vi "m1m3_getEvent_InclinometerSensorWarning.vi"(8 "error in (no error)":errorcluster, 11 "logevent_InclinometerSensorWarning_Ctl":T1) -> (0 "error out":errorcluster, 2 "function return":i32, 3 "logevent_InclinometerSensorWarning_Ctl out":T1)   [LabVIEW 2016, in "SALLV_m1m3.lvlib"]
doc: "int m1m3_shm_getEvent_InclinometerSensorWarningLV(m1m3_logevent_InclinometerSensorWarningLV *logevent_InclinometerSensorWarning_Ctl );"
uses:
  SALLV_m1m3.lvlib
  DataTypes/logevent_InclinometerSensorWarning.ctl
  SALLV_m1m3.so
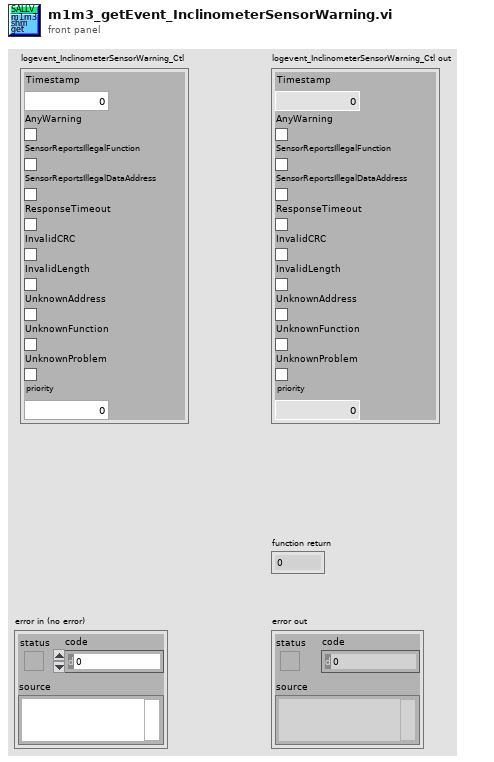
[diagram p1: front panel]
types:
  T1 = typedef "SALLV_m1m3.lvlib/logevent_InclinometerSensorWarning.ctl" = cluster{"Timestamp":dbl, "AnyWarning":bool, "SensorReportsIllegalFunction":bool, "SensorReportsIllegalDataAddress":bool, "ResponseTimeout":bool, "InvalidCRC":bool, "InvalidLength":bool, "UnknownAddress":bool, "UnknownFunction":bool, "UnknownProblem":bool, "priority":i32}
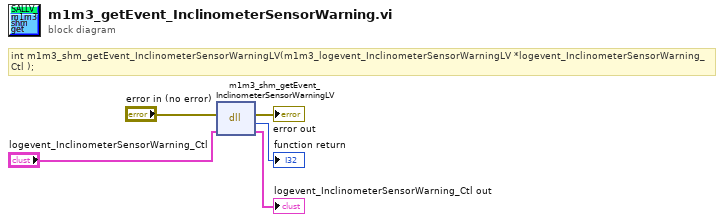
[diagram p0: block diagram]
diagram:
  # "int m1m3_shm_getEvent_InclinometerSensorWarningLV(m1m3_logevent_InclinometerSensorWarningLV *logevent_InclinometerSensorWarning_Ctl );"
  n1 = dll-call lib="opt/CODE/SALLV_m1m3/SALLV_m1m3.*" fn="m1m3_shm_getEvent_InclinometerSensorWarningLV"(error in="error in (no error)", "logevent_InclinometerSensorWarning_Ctl"="logevent_InclinometerSensorWarning_Ctl") -> (error out=→"error out":errorcluster, →"function return":i32, "logevent_InclinometerSensorWarning_Ctl"=→"logevent_InclinometerSensorWarning_Ctl out":T1)  [unwired: 2 in, 1 out]
